vi "Center Wheel.vi"(8 "Force strafe":bool, 10 "Center Wheel Value":dbl, 11 "MotorControlDevRef":T1={"DeviceStatus"={"status"=FALSE, "code"=0, "source"=""}, "Type"=enum."PWM", "PWM"={"Controller"=enum."Controller 1", "PWM Channel"=enum."Invalid", "DeadBand"={"Name"="", "maxPositivePwm"=0, "minPositivePwm"=0, "centerPwm"=0, "maxNegativePwm"=0, "minNegativePwm"=0, "angularRange"=0}}, "CAN"={"Device Number"=0, "Control Mode"=enum."Percent VBus", "Semaphore"=refnum, "Max Vout"=12.0, "TalonSRX Control Mode"=enum."Percent VBus"}, "Invert"=FALSE, "TransformRef"=refnum, "InvTransformRef"=refnum}) -> (1 "Wheel Down":bool, 2 "X Out":dbl, 3 "MotorControlDevRef 2":T1={"DeviceStatus"={"status"=FALSE, "code"=0, "source"=""}, "Type"=enum."PWM", "PWM"={"Controller"=enum."Controller 1", "PWM Channel"=enum."Invalid", "DeadBand"={"Name"="", "maxPositivePwm"=0, "minPositivePwm"=0, "centerPwm"=0, "maxNegativePwm"=0, "minNegativePwm"=0, "angularRange"=0}}, "CAN"={"Device Number"=0, "Control Mode"=enum."Percent VBus", "Semaphore"=refnum, "Max Vout"=12.0, "TalonSRX Control Mode"=enum."Percent VBus"}, "Invert"=FALSE, "TransformRef"=refnum, "InvTransformRef"=refnum})   [LabVIEW 2014]
uses:
  <vilib>/Rock Robotics/WPI/MotorControl/WPI_MotorControlDeviceRef.ctl
  <vilib>/Rock Robotics/WPI/MotorControl/WPI_MotorControlType.ctl
  <vilib>/Rock Robotics/SystemInterfaces/Typedef/FPGA_TypedefDigitalModule.ctl
  <vilib>/Rock Robotics/SystemInterfaces/DIO/FPGA_DIOPWMChannel.ctl
  <vilib>/Rock Robotics/WPI/PWM/WPI_PWMDeadband.ctl
  <vilib>/Rock Robotics/WPI/CAN/Jaguar/SubVIs/WPI_CANJaguar_ControlMode.ctl
  <vilib>/Rock Robotics/WPI/CAN/TalonSRX/WPI_CANTalonSRX_APIControlMode.ctl
  <vilib>/Rock Robotics/WPI/PWM/WPI_PWMTransform_ConPane.ctl
  <vilib>/Rock Robotics/WPI/Solenoid/Deprecated/WPI_SolenoidSetBool.vi
  Robot Global Data.vi
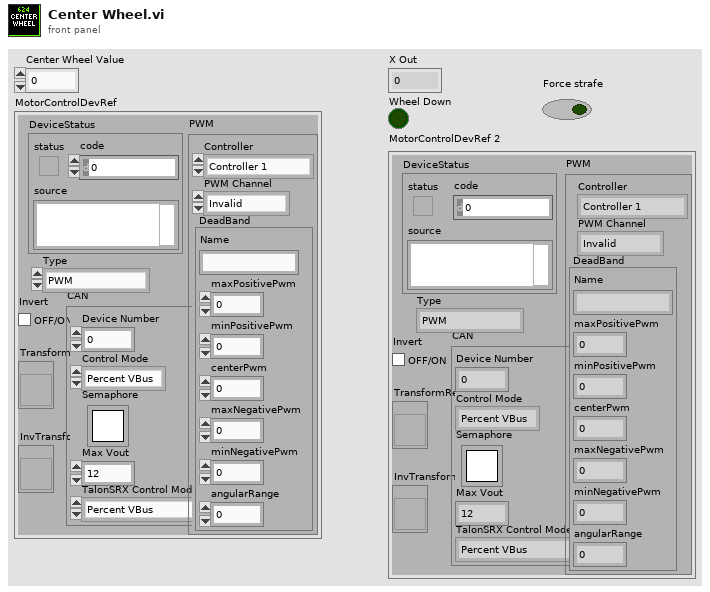
[diagram p1: front panel]
types:
  T1 = typedef "WPI_MotorControlDeviceRef.ctl" = cluster{"DeviceStatus":errorcluster, "Type":T2, "PWM":cluster{"Controller":T3, "PWM Channel":T4, "DeadBand":T5}, "CAN":cluster{"Device Number":u8, "Control Mode":T6, "Semaphore":T7, "Max Vout":dbl, "TalonSRX Control Mode":T8}, "Invert":bool, "TransformRef":T9, "InvTransformRef":T9}
  T2 = typedef "WPI_MotorControlType.ctl" = enum16{"PWM", "CAN", "CANTalonSRX"}
  T3 = typedef "FPGA_TypedefDigitalModule.ctl" = enum16{"Controller 1"}
  T4 = typedef "FPGA_DIOPWMChannel.ctl" = enum8{"PWM 0", "PWM 1", "PWM 2", "PWM 3", "PWM 4", "PWM 5", "PWM 6", "PWM 7", "PWM 8", "PWM 9", "PWM MXP 0", "PWM MXP 1", "PWM MXP 2", "PWM MXP 3", "PWM MXP 4", "PWM MXP 5", "PWM MXP 6", "PWM MXP 7", "PWM MXP 8", "PWM MXP 9", "Invalid"}
  T5 = typedef "WPI_PWMDeadband.ctl" = cluster{"Name":string, "maxPositivePwm":i32, "minPositivePwm":i32, "centerPwm":i32, "maxNegativePwm":i32, "minNegativePwm":i32, "angularRange":u16}
  T6 = typedef "WPI_CANJaguar_ControlMode.ctl" = enum8{"Percent VBus", "Current", "Speed", "Position", "Voltage"}
  T7 = typedef "Semaphore RefNum" = refnum<k1>
  T8 = typedef "WPI_CANTalonSRX_APIControlMode.ctl" = enum8{"Percent VBus", "Speed", "Position", "Slave", "Unchanged / Invalid"}
  T9 = typedef "WPI_PWMTransform_ConPane.ctl" = refnum<vi>
  T10 = typedef "Dashboard Control Data.ctl" = cluster{"Cam Exposure":dbl, "Go to angle":dbl, "Steer PID Gains":cluster{"proportional gain (Kc)":dbl, "integral time (Ti, min)":dbl, "derivative time (Td, min)":dbl}, "Steer PID output Range":cluster{"output high":dbl, "output low":dbl}, "Pressure m \nValue":dbl, "Pressure b \nValue":dbl, "Roller Command Cluster ":T11, "Elevator":T12, "Encoder Control":T14, "Auton Settings":cluster{"Drive Dist Window Size":dbl}, "Drivetrain Settings":T15}
  T11 = typedef "Roller Control.ctl" = cluster{"Intake Speed":dbl, "Turn In Speed":dbl, "Unload Speed":dbl, "Turn Out Speed":dbl, "Ping Align Tolerance":dbl, "Tote Range Threshold":dbl, "Right Pot 0":dbl, "Pot Threshold":dbl, "Left Pot 0":dbl, "Manual 0s?":bool, "Right Pot Scale":dbl, "Left Pot Scale":dbl, "0 wait time":i32, "Zero Pots":bool, "Min Elevator Height":dbl, "Eject Time":dbl, "Eject US Threshold":dbl, "Anti-Twitch Time":u32, "Ping Caring Threshold":dbl, "Pot Diff Threshold":dbl, "Pinch Sustain":u32, "Absorb Give Up Threshold":dbl, "Untip In Threshold":dbl, "Untip Grab Range":dbl, "Ultrasonic Hold Time":u32, "Landscape Absorb Time":u32, "Pot Use Wait Time":u32, "Can Turn Stop Range":dbl, "Ignore Pressure":bool}
  T12 = typedef "Elevator DB Control.ctl" = cluster{"PID Output Range":cluster{"output high":dbl, "output low":dbl}, "PID gains":cluster{"proportional gain (Kc)":dbl, "integral time (Ti, min)":dbl, "derivative time (Td, min)":dbl}, "Height Tolerance":sgl, " Encoder Constant":dbl, "Safe Mode Max Speed":sgl, "Eject Time":sgl, "Zeroing Speed":sgl, "Presets":T13, "Ping Detect Threshold":sgl, "Trashcan Detect Threshold":sgl, "Zero Filter Time":dbl, "Stabilizer Open Time":dbl, "Zero Creep Speed":dbl, "Max Current":dbl, "Current Trip Time":dbl, "Abort Pitch":dbl}
  T13 = typedef "Elevator Presets.ctl" = cluster{"Pickup 2 w/ Tote":sgl, "Pickup 2 w/ Trashcan":sgl, "Pickup 3 w/ Tote":sgl, "Pickup 3 w/ Trashcan":sgl, "Bottom":sgl, "Pickup 1 w/ Tote":sgl, "Pickup Trashcan":sgl, "Pickup 1 w/ Trashcan":sgl, "Eject":sgl, "Hold Low":sgl, "Step add height":sgl, "Store Trashcan 1":sgl, "Store Trashcan 2":sgl, "Store Trashcan 3":sgl, "6 Tote Max":sgl, "5 Tote Max":sgl, "Untip Lift":dbl, "Drop Stack":dbl, "Pickup 1 Empty":dbl, "Pickup 2 Empty":dbl, "Pickup 3 Empty":dbl, "4 Tote Max":dbl, "HP Load Hold":dbl, "HP Load Drop":dbl, "HP Load Finger":dbl, "HP Load Hold Can":dbl, "Stop store open stab":dbl}
  T14 = typedef "Encoder Control.ctl" = cluster{"Left Tick Constant":dbl, "Right Tick Constant":dbl, "Center Tick Constant":dbl, "Reset?":bool, "Y Dist":cluster{"PID gains":cluster{"proportional gain (Kc)":dbl, "integral time (Ti, min)":dbl, "derivative time (Td, min)":dbl}}, "X Dist":cluster{"PID gains":cluster{"proportional gain (Kc)":dbl, "integral time (Ti, min)":dbl, "derivative time (Td, min)":dbl}}, "Y Stop Thresh":dbl, "Y Stop Speed":dbl, "X Stop Thresh":dbl, "X Stop Speed":dbl}
  T15 = typedef "Drivetrain Settings.ctl" = cluster{"Gyro Tolerance":dbl, "Strafe Correct max steer":dbl, "Strafe Timer Wait":dbl, "Throttle Ramp (ms)":dbl, "Strafe Ramp (ms)":dbl, "Angular rate compensation":bool, "Throttle to Rate Scale":dbl, "Rate compensation gain":dbl}
  T16 = typedef "WPI_SolenoidDevRef.ctl" = cluster{"DevStatus":errorcluster, "Pneumatics Control Module":u8, "Forward Solenoid Channel":T17, "Reverse Solenoid Channel":T17}
  T17 = typedef "WPI_SolenoidChannel.ctl" = enum8{"Solenoid 0", "Solenoid 1", "Solenoid 2", "Solenoid 3", "Solenoid 4", "Solenoid 5", "Solenoid 6", "Solenoid 7", "Invalid"}
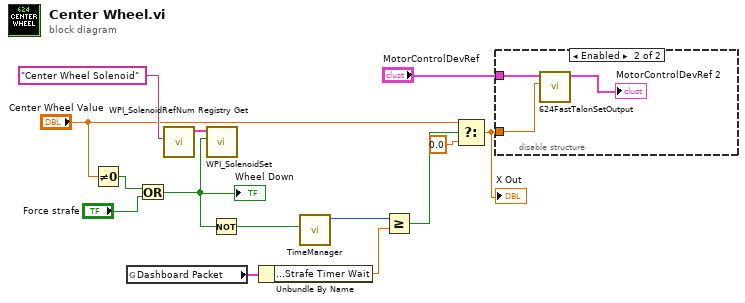
[diagram p0: block diagram]
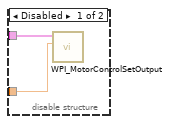
[diagram p2: hidden frame]
diagram:
  n1 = Not Equal To 0?(x="Center Wheel Value") -> (x != 0?=w3:bool)
  n2 = global read "Robot Global Data.vi" "Dashboard Packet"() -> (w12:T10)
  n3 = Or(x=w3, y="Force strafe") -> (x .or. y?=w1:bool)
  "Wheel Down" <- w1
  n4 = call <vilib>:"WPI_SolenoidRefNum Registry Get.vi"("refnum name"="Center Wheel Solenoid") -> ("SolenoidDevRef"=w13:T16)  [unwired: 9 in, 1 out]
  n5 = call-poly <vilib>:"WPI_SolenoidSet.vi"("Value"=w1, "SolenoidDevRef"=w13) -> ()  [unwired: 8 in, 2 out]
  n6 = Not(x=w1) -> (.not. x?=w5:bool)
  n7 = Unbundle By Name(w12) -> ("Drivetrain Settings.Strafe Timer Wait"=w11:dbl)
  n8 = call "TimeManager.vi"("Reset?"=w5) -> ("Time Since Reset"=w10:u32)  [unwired: 9 in, 1 out]
  n9 = Greater Or Equal?(x=w10, y=w11) -> (x >= y?=w9:bool)
  n10 = Select(t="Center Wheel Value", s=w9, f=0.0) -> (s? t:f=w6:dbl)
  "X Out" <- w6
  n11 = disable-structure shown="Enabled" {
    disable-tunnel: "MotorControlDevRef" -> [w16 w19]
    disable-tunnel: w6 -> [w15 w18]
    frame Disabled {
      n12 = call <vilib>:"WPI_MotorControlSetOutput.vi"("Output"=w15, "MotorControlDevRef"=w16) -> ()  [unwired: 7 in, 3 out]
    }
    frame Enabled {
      n13 = call "624FastTalonSetOutput.vi"("Output"=w18, "MotorControlDevRef"=w19) -> ("MotorControlDevRef"=→"MotorControlDevRef 2":T1)  [unwired: 8 in, 1 out]
    }
  }
